vi "Measurement_input_panel.vi"(0 "OK":T4, 2 "setup":T5, 5 "Setup filename":string) -> (11 "Setup filename out":string, 12 "Analysis Info cluster":T8[](array[typedef])=[{"Colour"=0, "Inst type"=enum."Pitot-static tube", "Inst name"="Manometer voltage", "Symbol"="U", "Code name"="", "Extra Info"="U", "Inst Array"=enum."PWA", "Extra Titles"=[], "Extra Values"=[], "U"=0.0, "u^2"=0.0, "u^3"=0.0, "u^4"=0.0, "Skew_u"=0.0, "Kurt_u"=0.0, "Sd Error in Mean"=0.0, "% u'/U"=0.0, "X"=0.0, "Y"=0.0, "Z"=0.0, "Timescale integral to 25%"=0.0, "Sd Error in Variance"=0.0, "Calib File"=path "", "Calib Constants"=[], "Output Position"=FALSE, "Full Stats"=FALSE, "Av Sampling Rate"=0.0, "Av No of Samples"=0.0, "Total Meas Time (s)"=0.0, "ADAM Ch Name"=""}, {"Colour"=0, "Inst type"=enum."Pitot-static tube", "Inst name"="Manometer voltage", "Symbol"="U", "Code name"="", "Extra Info"="U", "Inst Array"=enum."PWA", "Extra Titles"=[], "Extra Values"=[], "U"=0.0, "u^2"=0.0, "u^3"=0.0, "u^4"=0.0, "Skew_u"=0.0, "Kurt_u"=0.0, "Sd Error in Mean"=0.0, "% u'/U"=0.0, "X"=0.0, "Y"=0.0, "Z"=0.0, "Timescale integral to 25%"=0.0, "Sd Error in Variance"=0.0, "Calib File"=path "", "Calib Constants"=[], "Output Position"=FALSE, "Full Stats"=FALSE, "Av Sampling Rate"=0.0, "Av No of Samples"=0.0, "Total Meas Time (s)"=0.0, "ADAM Ch Name"=""}, {"Colour"=0, "Inst type"=enum."Pitot-static tube", "Inst name"="Manometer voltage", "Symbol"="U", "Code name"="", "Extra Info"="U", "Inst Array"=enum."PWA", "Extra Titles"=[], "Extra Values"=[], "U"=0.0, "u^2"=0.0, "u^3"=0.0, "u^4"=0.0, "Skew_u"=0.0, "Kurt_u"=0.0, "Sd Error in Mean"=0.0, "% u'/U"=0.0, "X"=0.0, "Y"=0.0, "Z"=0.0, "Timescale integral to 25%"=0.0, "Sd Error in Variance"=0.0, "Calib File"=path "", "Calib Constants"=[], "Output Position"=FALSE, "Full Stats"=FALSE, "Av Sampling Rate"=0.0, "Av No of Samples"=0.0, "Total Meas Time (s)"=0.0, "ADAM Ch Name"=""}] {"Sd Error in Variance" format="%.2f"; "Skew_u" format="%.2f"; "% u'/U" format="%.2f"; "Sd Error in Mean" format="%.2f"; "Kurt_u" format="%.2f"; "u^4" format="%.2f"; "u^3" format="%.2f"; "U" format="%.2f"; "u^2" format="%.2f"})   [LabVIEW 2013]
uses:
  Controls/Ch_and_spans_choices.ctl
  Controls/Inst_type.ctl
  Controls/Analysis_info_cluster.ctl
  Controls/Instrument_Array.ctl
  Controls/LDA_Setup.ctl
  Controls/Setup.ctl
  Controls/ok_button.ctl
  Controls/Trigger_Mode.ctl
  Controls/PWA_Data.ctl
  File/Setup_Filetype.ctl
  Controls/Post_Process.ctl
  Controls/App_Global.ctl
  Controls/Ch_and_Spans.ctl
  Globals/Meas_global.vi
  Globals/Trav_pos_global.vi
  Globals/LDA_meas_global_1.vi
  Globals/Preference_global.vi
panel:
  in  "Acquisition Plug in":u16(ring) items=["ADAM_Server_Channels.vi", "Channels_and_Index.ctl", "DataTranslation.vi", "DT_With_Multiplexer.vi", "LDA_IP.vi", "NI-DAQmx.vi", "Simulate_kernal.vi"]
  in  "Select Duplicate Channels":bool
  in  "PWA Data":T1
  out "Inst type":T2
  in  "Edit temp and Press":bool
  out "Abs Press (mbar)":dbl=1013.0 format="%.1f"
  out "Temp (deg C)":dbl=21.0 format="%.1f"
  in  "Trigger mode":T3
  in  "Select Plug Ins":bool
  in  "Sync Delay Time (ms)":dbl=24.0 format="%.2f"
  out "XW Present?":bool
  out "Read Setup File?":bool
  out "Setup Paths":string[](array[string])
  in  "Select Local ADAM Channels":bool
  in  "stop":bool
  out "Notes":string
  in  "Setup filename selector":u16(ring) items=["Current_Setup.xls"]
  in  "Synchronise Analogue channels with LDA":bool
  in  "LDA set up":T6={"dimensions"=enum."2D", "Analogue Freq Multiplier"=0.1} {"Analogue Freq Multiplier" min=0.1 max=100.0 format="%_5g"}
  in  "LDA data":enum16{"No LDA data", "Take LDA data"}(ring)=enum."Take LDA data"
  in  "Cross wire":T7(ring)
  in  "No of Analogue inst":i32=1
  in  "Ch & spans choices":T10[](array[typedef]) {"D" format="%.2f"; "Ch No" min=0; "low limit" min=-10 max=10 format="%.2f"; "high limit" min=-10 max=10 format="%.2f"}
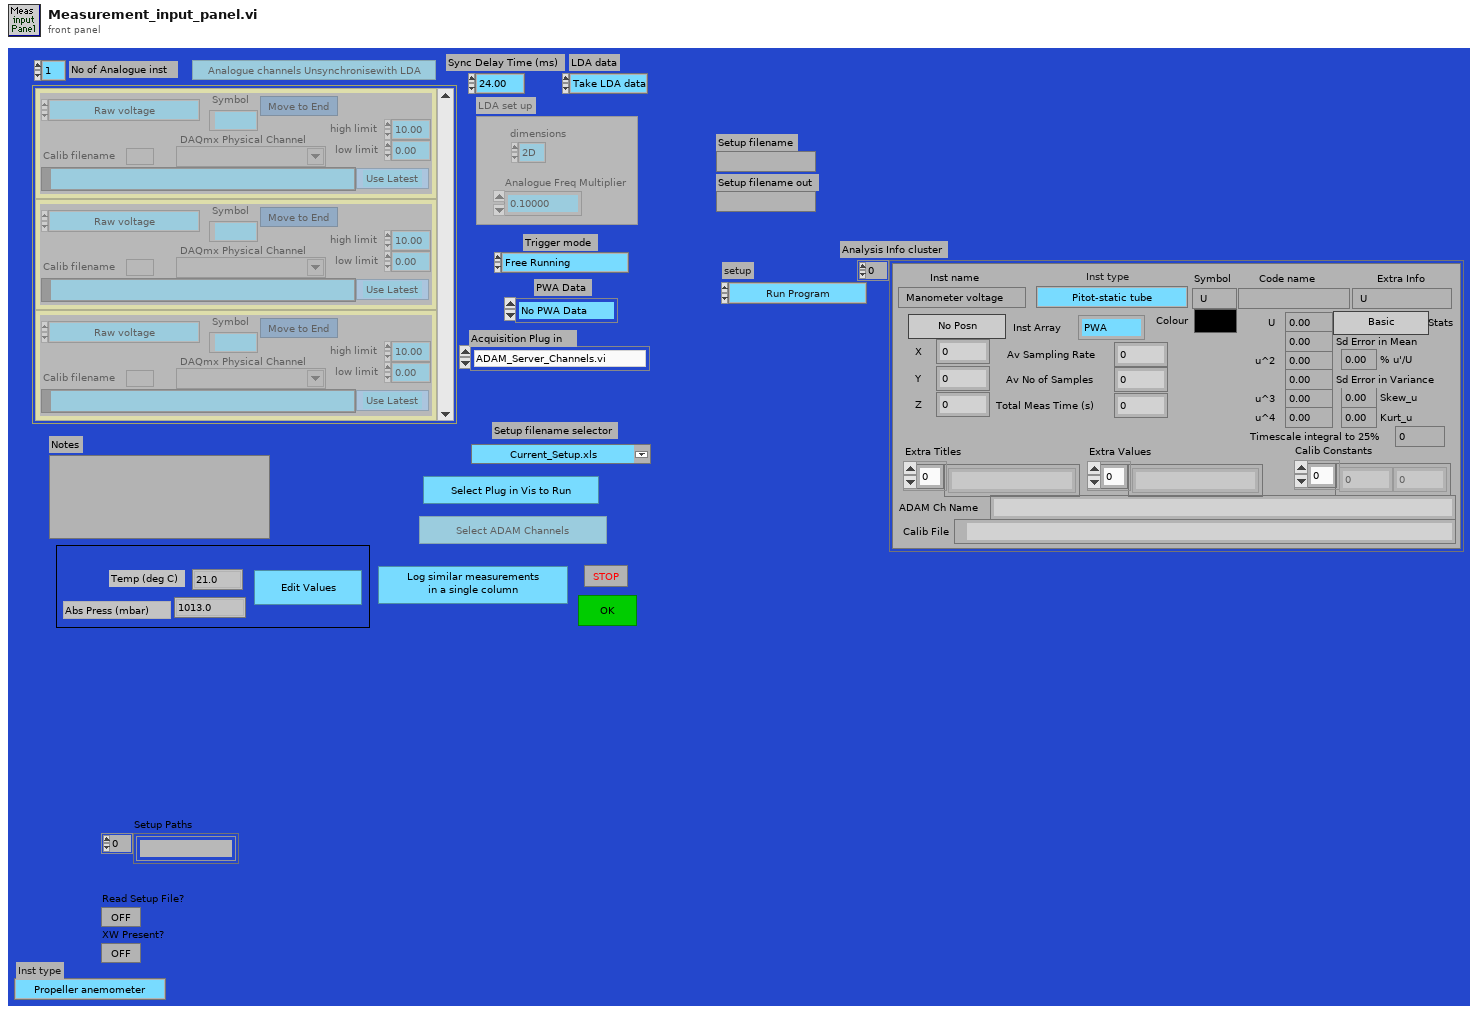
[diagram p1: front panel]
types:
  T1 = typedef "PWA_Data.ctl" = enum16{"No PWA Data", "One Ch PWA"}
  T2 = typedef "Inst_type.ctl" = enum16{"Propeller anemometer", "Raw voltage", "Pressure Transducer", "Pitot-static tube", "Preston tube", "Hot wire", "Cross wire 1", "Cross wire 2", "Generic Linear", "Generic Polynomial", "Generic BackPoly", "Fast FID", "Thermocouple", "Cold wire", "Pulsed Wire", "LDA Vel", "LDA Tran time", "LDA Arr time"}
  T3 = typedef "Trigger_Mode.ctl" = enum16{"Free Running", "Start on Trigger", "Trigger Every Block", "Trigger Every Sample"}
  T4 = typedef "ok_button.ctl" = bool
  T5 = typedef "Setup.ctl" = enum16{"Run Program", "Show Setup", "Save Current Setup", "Setup Front Panel"}
  T6 = typedef "LDA_Setup.ctl" = cluster{"dimensions":enum16{"1D", "2D"}, "Analogue Freq Multiplier":dbl}
  T7 = enum16{"2nd component as calculated", "2nd component multipled by -1"}
  T8 = typedef "Analysis_info_cluster.ctl" = cluster{"Colour":u32, "Inst type":T2, "Inst name":string, "Symbol":string, "Code name":string, "Extra Info":string, "Inst Array":T9, "Extra Titles":string[], "Extra Values":string[], "U":dbl, "u^2":dbl, "u^3":dbl, "u^4":dbl, "Skew_u":dbl, "Kurt_u":dbl, "Sd Error in Mean":dbl, "% u'/U":dbl, "X":dbl, "Y":dbl, "Z":dbl, "Timescale integral to 25%":dbl, "Sd Error in Variance":dbl, "Calib File":path, "Calib Constants":dbl[], "Output Position":bool, "Full Stats":bool, "Av Sampling Rate":dbl, "Av No of Samples":dbl, "Total Meas Time (s)":dbl, "ADAM Ch Name":string}
  T9 = typedef "Instrument_Array.ctl" = enum16{"PWA", "LDA", "Analogue"}
  T10 = typedef "Ch_and_spans_choices.ctl" = cluster{"high limit":sgl, "low limit":sgl, "Ch No":i16, "Calib filename":path, "Inst type":T2, "Symbol":string, "Move channel":bool, "Use Latest":bool, "D":dbl, "Ch Name":string, "DAQmx Physical Channel":tag}
  T11 = typedef "Post_Process.ctl" = enum16{"Take New Data", "Post Process Raw Data File"}
  T12 = typedef "Setup_Filetype.ctl" = enum16{"Measurement Setups", "Calibration Setups", "General", "Results File Plotter Setups", "Speed Calib Tweaks"}
  T13 = typedef "App_Global.ctl" = enum16{"Read Global", "Write to Global", "Initialise Array"}
  T14 = typedef "Ch_and_Spans.ctl" = cluster{"high limit (10V)":sgl, "low limit (-10V)":sgl, "Ch No":i16, "Var name":string, "Use Latest Calib":bool, "DAQmx Chan":tag}
  T15 = enum16{"Zero or one", "One", "Zero or more", "One or more"}
  T16 = typedef "Traverse_cluster.ctl" = cluster{"Start X":dbl, "Start Y":dbl, "Start Z":dbl, "End X":dbl, "End Y":dbl, "End Z":dbl, "No. of pts.":i32, "Spacing":T17, "Filename":path, "Tunnel Speed":dbl, "Averaging time (min)":dbl, "Extra Commands":string, "Specific Arguments":string, "Emission Rate (l/min)":dbl, "Trace Gas Concentration (%)":dbl, "Density Ratio":string, "Comments":string, "Row No":i32, "Row Type Selector":T18, "Completion time":string, "Row Duration (mins)":dbl, "No. of Valid pts.":i32, "Meas Setup File":string}
  T17 = typedef "Spacing.ctl" = enum16{"Linear", "Log", "Gauss", "Specified", "N/A"}
  T18 = typedef "Multi_run_mode.ctl" = enum16{"Move Traverse Only", "Set Tunnel Speed Only", "Set Source Only", "Set Measurement Conditions", "Single Measurement", "Vertical Profile", "Lateral Profile", "Longitudinal Profile", "Explore Volume", "Multi-Axis Profile", "Auto Calibrate", "Meas Fast FID Bkgnd", "Check Beam Power", "Scanning Valve Measurement", "Run VI Named:", "Set ADAM Ch", "Wait (minutes)", "Send Message", "Synchronize With:", "Fall Back to this Row", "Turn Off Row Repeating", "Blank Row", "Traverse 3D Volume"}
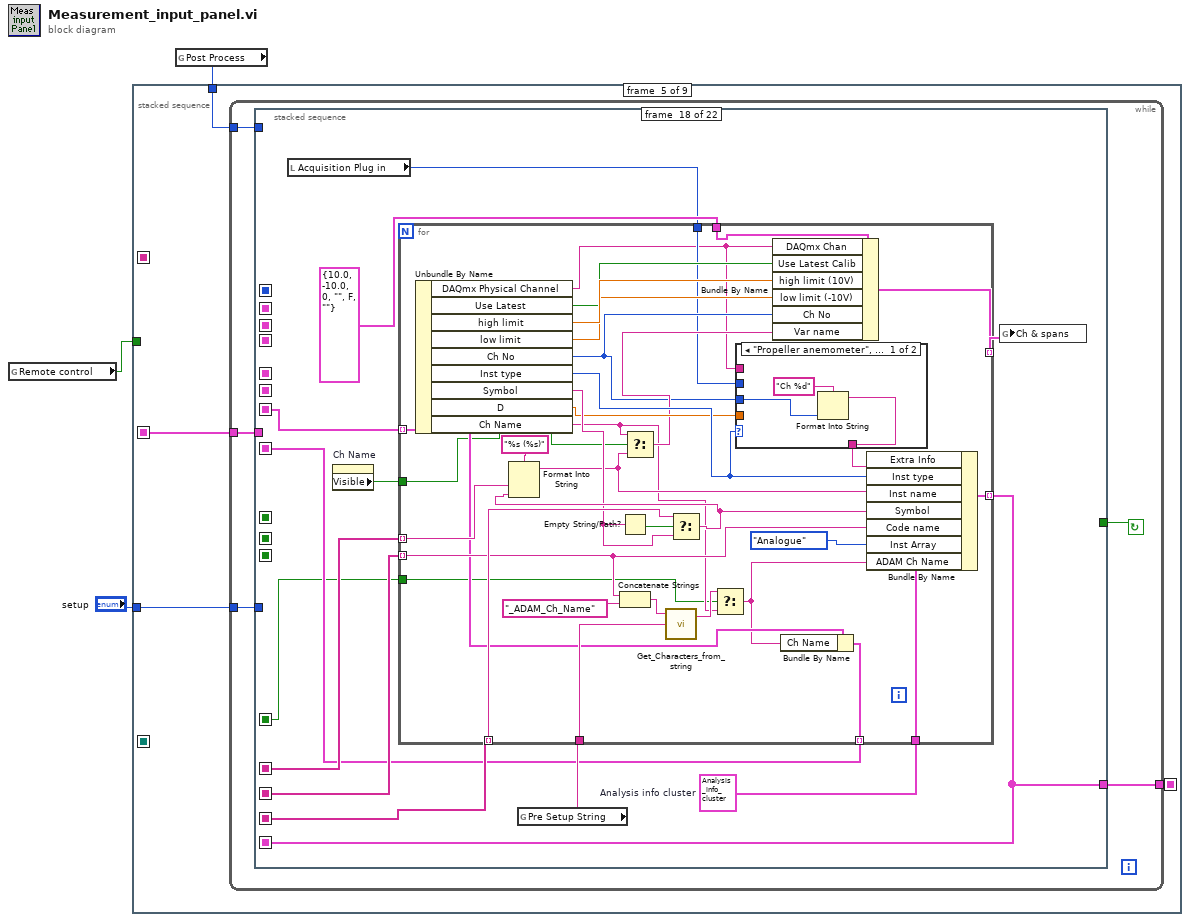
[diagram p0: block diagram]
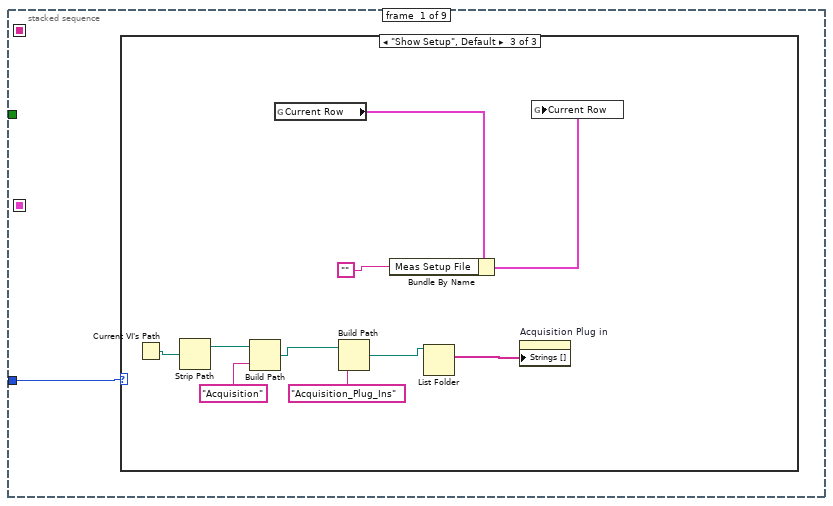
[diagram p2: hidden frame]
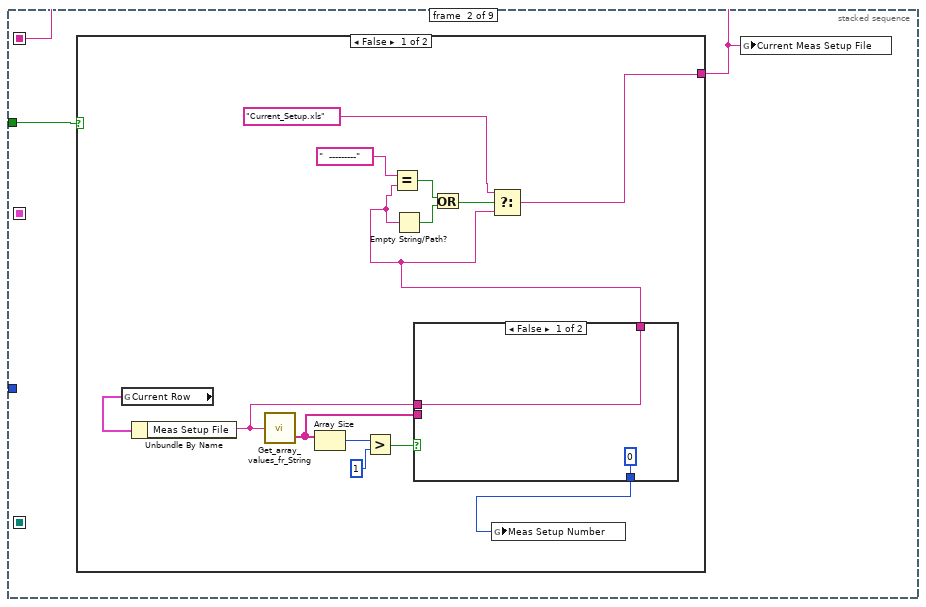
[diagram p5: hidden frame]
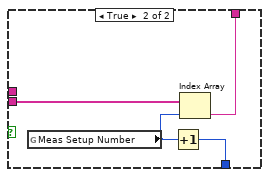
[diagram p6: hidden frame]
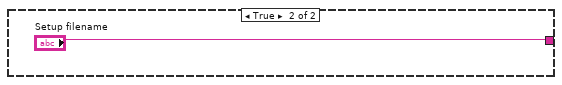
[diagram p7: hidden frame]
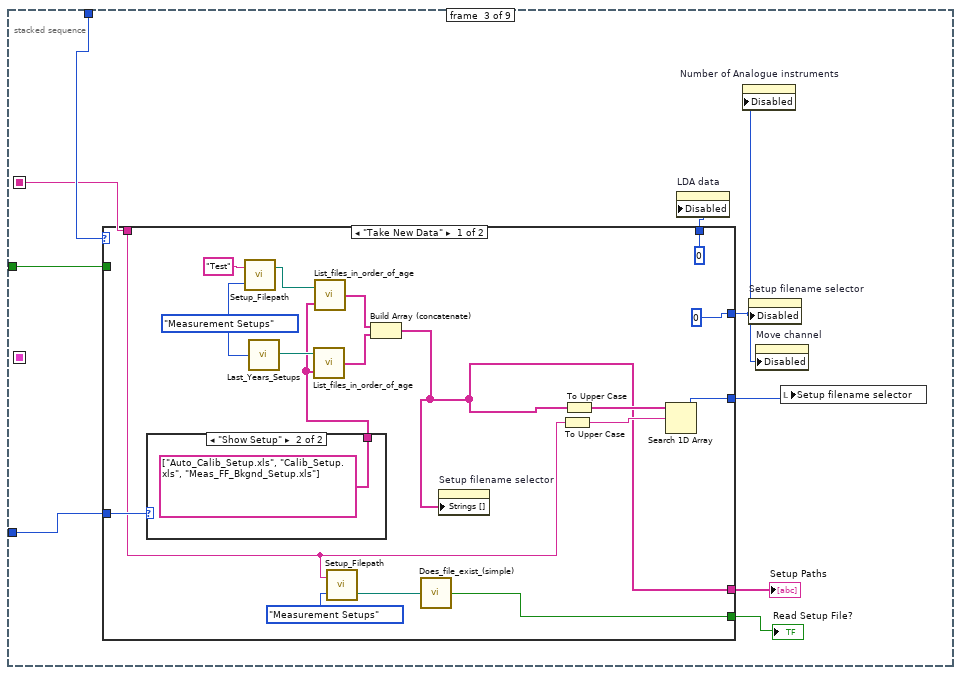
[diagram p8: hidden frame]
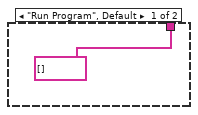
[diagram p9: hidden frame]
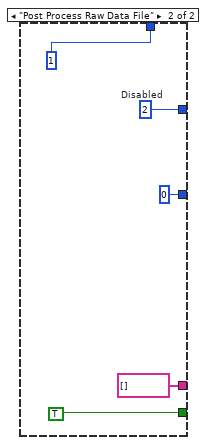
[diagram p10: hidden frame]
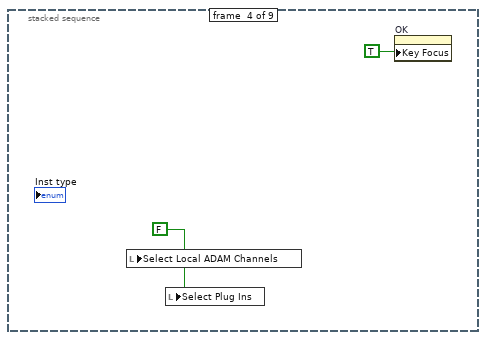
[diagram p11: hidden frame]
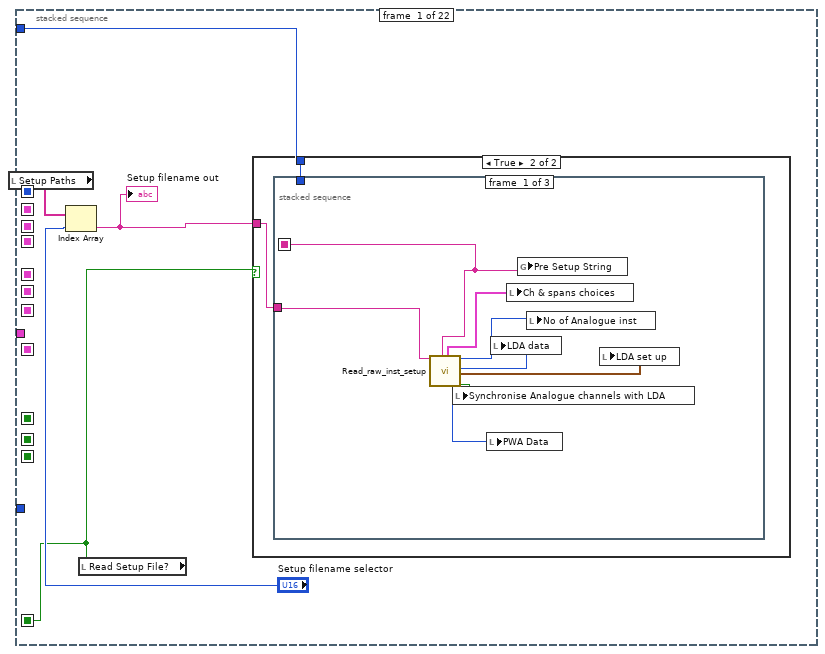
[diagram p12: hidden frame]
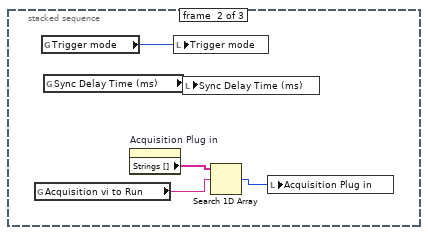
[diagram p14: hidden frame]
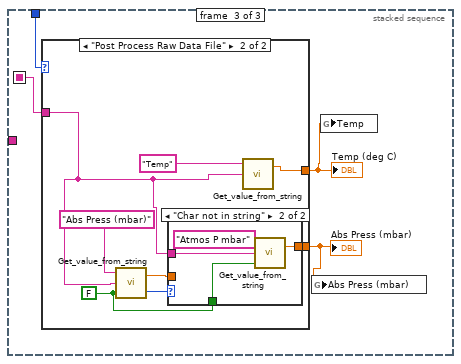
[diagram p15: hidden frame]
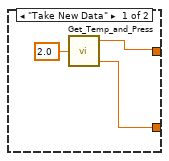
[diagram p16: hidden frame]
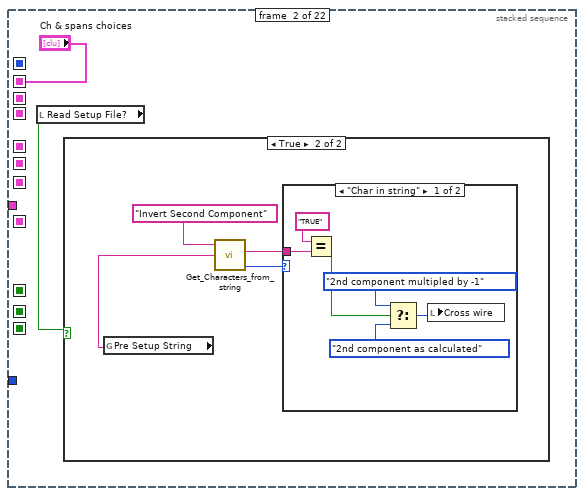
[diagram p18: hidden frame]
diagram:
  n1 = global read "Meas_global.vi" "Remote control"() -> (w1:bool)
  n2 = global read "Meas_global.vi" "Post Process"() -> (w3:T11)
  n3 = stacked-sequence {
    seq-local: [_ _ _ _ w77 _ _ _ _] -> [_ _ _ _ _ _ w720 w821 _]
    seq-local: [_ w15 _ _ _ _ _ _ _] -> [_ _ w38 _ _ _ w719 _ _]
    seq-local: [_ _ _ _ w74 _ _ _ _] -> [_ _ _ _ _ _ _ _ w873]
    seq-local: [_ _ _ _ _ _ _ w820 _] -> [_ _ _ _ _ _ _ _ w872]
    tunnel: w3 -> [_ _ w46 _ w76 _ _ w822 _]
    tunnel: "setup" -> [w4 _ w40 _ w75 _ w721 _ _]
    tunnel: w1 -> [_ w16 w39 _ _ _ _ _ _]
    frame #0 {
      n4 = case shown="\"Show Setup\", Default" w4 {
        frame "Run Program" {
        }
        frame "Setup Front Panel" {
        }
        frame "Show Setup", Default {
          n5 = Current VI's Path() -> (path=w11:path)
          n6 = Strip Path(path=w11) -> (stripped path=w10:path)  [unwired: 1 out]
          n7 = Build Path(base path=w10, name or relative path="Acquisition") -> (appended path=w7:path)
          n8 = global read "Trav_pos_global.vi" "Current Row"() -> (w14:T16)
          n9 = Build Path(base path=w7, name or relative path="Acquisition_Plug_Ins") -> (appended path=w6:path)
          n10 = Bundle By Name(cluster=w14, "Meas Setup File"="") -> (w13:T16)
          n11 = List Folder(path=w6) -> (filenames=w5:string[])  [unwired: 3 in, 3 out]
          n12 = property on="Acquisition Plug in" class="Ring (strict)"("Strings []"=w5) -> ()  [unwired: 2 in, 2 out]
          n13 = global write "Trav_pos_global.vi" "Current Row"(w13) -> ()
        }
      }
    }
    frame #1 {
      n14 = case shown="False" w16 {
        tunnel: [w29 "Setup filename"] -> w15
        frame False {
          n15 = global read "Trav_pos_global.vi" "Current Row"() -> (w25:T16)
          n16 = Unbundle By Name(w25) -> ("Meas Setup File"=w19:string)
          n17 = call "Get_array_values_fr_String.vi"("String Value"=w19) -> ("String array"=w18:string[])  [unwired: 1 out]
          n18 = Array Size(array=w18) -> (size(s)=w23:i32)
          n19 = Greater?(x=w23, y=1) -> (0:w21:bool)
          n20 = case shown="False" w21 {
            tunnel: [w32 w35] -> w20
            tunnel: w19 -> [w32 _]
            tunnel: w18 -> [_ w36]
            tunnel: [0 w33] -> w17
            frame False {
            }
            frame True {
              n21 = global read "Trav_pos_global.vi" "Meas Setup Number"() -> (w34:i32)
              n22 = Increment(x=w34) -> (x+1=w33:i32)
              n23 = Index Array(array=w36, index=w34) -> (element=w35:string)
            }
          }
          n24 = Equal?(x="  ---------" ("f"), y=w20) -> (x = y?=w28:bool)
          n25 = Empty String/Path?(string/path=w20) -> (empty?=w27:bool)
          n26 = Or(x=w28, y=w27) -> (x .or. y?=w24:bool)
          n27 = Select(t="Current_Setup.xls", s=w24, f=w20) -> (s? t:f=w29:string)
          n28 = global write "Trav_pos_global.vi" "Meas Setup Number"(w17) -> ()
        }
        frame True {
        }
      }
      n29 = global write "Trav_pos_global.vi" "Current Meas Setup File"(w15) -> ()
    }
    frame #2 {
      n30 = case shown="\"Take New Data\"" w46 {
        tunnel: [w47 string[] []] -> w42
        tunnel: [w60 TRUE ("exists")] -> w41
        tunnel: [u8 0 ("Disabled") w68] -> w43
        tunnel: [u8 0 ("Disabled") u8 1 ("Disabled")] -> w45
        tunnel: w38 -> [w56 _]
        tunnel: [w63 0 ("index of element")] -> w44
        tunnel: w40 -> [w58 _]
        tunnel: w39 -> [_ _]
        frame "Take New Data" {
          w50 = Setup_Filetype."Measurement Setups" ("Setup File Type")
          n31 = case shown="\"Show Setup\"" w58 {
            tunnel: [string[] [] ("file names") string[] ["Auto_Calib_Setup.xls", "Calib_Setup.xls", "Meas_FF_Bkgnd_Setup.xls"] ("file names")] -> w48
            frame "Run Program", Default {
            }
            frame "Show Setup" {
            }
          }
          n32 = call "Setup_Filepath.vi"("Setup File Type"=w50, "Filename in"="Test") -> ("Directory"=w51:path)  [unwired: 1 out]
          n33 = call "Last_Years_Setups.vi"("Setup File Type"=w50) -> ("Directory"=w49:path)
          n34 = call "List_files_in_order_of_age.vi"("Files to Hide"=w48, "Folder"=w49) -> ("file names"=w53:string[])
          n35 = call "List_files_in_order_of_age.vi"("Files to Hide"=w48, "Folder"=w51) -> ("file names"=w52:string[])
          n36 = call "Setup_Filepath.vi"("Setup File Type"=Setup_Filetype."Measurement Setups", "Filename in"=w56) -> ("Filename Out"=w55:path)  [unwired: 1 out]
          n37 = Build Array (concatenate)(w52, w53) -> (w47:string[])
          n38 = call "Does_file_exist_(simple).vi"("Pathname"=w55) -> ("exists?"=w60:bool)
          n39 = property on="Setup filename selector" class="Ring (strict)"("Strings []"=w47) -> ()  [unwired: 2 in, 2 out]
          n40 = To Upper Case(1:w56) -> (0:w61:string)
          n41 = To Upper Case(1:w47) -> (0:w62:string[])
          n42 = Search 1D Array(1D array=w62, element=w61) -> (index of element=w63:i32)  [unwired: 1 out]
        }
        frame "Post Process Raw Data File" {
          w68 = u8 2  # Disabled
        }
      }
      "Setup Paths" <- w42
      "Read Setup File?" <- w41
      n43 = property on="LDA data" class="Enum (strict)"("Disabled"=w45) -> ()  [unwired: 2 in, 2 out]
      n44 = property on="Number of Analogue instruments" class="DigNum (strict)"("Disabled"=w43) -> ()  [unwired: 2 in, 2 out]
      n45 = property on="Setup filename selector" class="Ring (strict)"("Disabled"=w43) -> ()  [unwired: 2 in, 2 out]
      n46 = property on="Move channel" class="Bool (strict)"("Disabled"=w43) -> ()  [unwired: 2 in, 2 out]
      n47 = local write "Setup filename selector"(w44) -> ()
    }
    frame #3 {
      w73 = FALSE ("Select Local ADAM Channels")
      n48 = local write "Select Local ADAM Channels"(w73) -> ()
      n49 = local write "Select Plug Ins"(w73) -> ()
      n50 = property on="OK" class="Bool"("Key Focus"=TRUE) -> ()  [unwired: 2 in, 2 out]
    }
    frame #4 {
      n51 = while {
        tunnel: w75 -> [w79]
        tunnel: w76 -> [w80]
        tunnel: [w82] -> w77
        tunnel: [w78] -> w74
        stop <- w81 continue-if-true
        n52 = stacked-sequence {
          seq-local: [_ _ _ _ _ _ _ _ _ w242 _ _ _ _ _ _ _ _ _ _ _ _] -> [_ _ _ _ _ _ _ _ _ _ _ w305 w350 w415 _ _ _ _ _ _ _ _]
          seq-local: [_ _ _ _ w166 _ _ _ _ _ _ _ _ _ _ _ _ _ _ _ _ _] -> [_ _ _ _ _ _ w204 _ w238 w243 _ _ _ _ _ _ _ _ _ _ _ _]
          seq-local: [_ _ _ _ _ _ w209 _ _ _ _ _ _ _ _ _ _ _ _ _ _ _] -> [_ _ _ _ _ _ _ _ _ w244 _ _ _ _ _ _ _ _ _ _ _ _]
          seq-local: [_ _ _ _ _ _ _ _ _ _ _ w307 _ _ _ _ _ _ _ _ _ _] -> [_ _ _ _ _ _ _ _ _ _ _ _ w352 _ _ _ _ _ _ _ _ w685]
          seq-local: [_ _ _ _ _ _ _ _ _ _ _ _ _ _ w448 _ _ _ _ _ _ _] -> [_ _ _ _ _ _ _ _ _ _ _ _ _ _ _ w467 _ _ _ _ _ _]
          seq-local: [_ _ _ _ _ _ _ _ _ _ _ _ _ _ _ w463 _ _ _ _ _ _] -> [_ _ _ _ _ _ _ _ _ _ _ _ _ _ _ _ w491 w559 _ _ w661 w686]
          seq-local: [_ _ _ _ _ _ _ _ _ _ _ _ w356 _ _ _ _ _ _ _ _ _] -> [_ _ _ _ _ _ _ _ _ _ _ _ _ _ w445 _ _ _ _ _ _ _]
          seq-local: [_ _ _ _ _ _ _ _ _ _ _ _ _ w419 _ _ _ _ _ _ _ _] -> [_ _ _ _ _ _ _ _ _ _ _ _ _ _ w444 _ _ _ _ _ _ _]
          seq-local: [_ _ _ _ _ _ _ _ _ _ w302 _ _ _ _ _ _ _ _ _ _ _] -> [_ _ _ _ _ _ _ _ _ _ _ w306 w353 _ _ _ _ _ _ _ _ w684]
          seq-local: [_ _ _ _ _ _ _ _ _ _ _ _ _ _ _ _ w490 _ _ _ _ _] -> [_ _ _ _ _ _ _ _ _ _ _ _ _ _ _ _ _ w562 _ _ _ _]
          seq-local: [_ _ _ _ _ _ _ _ _ _ _ _ _ _ _ _ w489 _ _ _ _ _] -> [_ _ _ _ _ _ _ _ _ _ _ _ _ _ _ _ _ w561 _ _ _ _]
          seq-local: [_ _ _ _ _ _ _ _ _ _ _ _ _ _ _ _ w488 _ _ _ _ _] -> [_ _ _ _ _ _ _ _ _ _ _ _ _ _ _ _ _ w560 _ _ _ _]
          seq-local: [_ _ _ _ _ _ _ _ _ _ _ _ _ _ _ _ _ w558 _ _ _ _] -> [_ _ _ _ _ _ _ _ _ _ _ _ _ _ _ _ _ _ _ w611 _ _]
          seq-local: [_ "Ch & spans choices" _ _ _ _ _ _ _ _ _ _ _ _ _ _ _ _ _ _ _ _] -> [_ _ _ _ w155 _ _ _ _ _ _ _ _ _ _ _ _ _ w606 _ _ _]
          seq-local: [_ _ _ _ _ _ _ _ _ _ _ _ _ _ _ _ _ w556 _ _ _ _] -> [_ _ _ _ _ _ _ _ _ _ _ _ _ _ _ _ _ _ w605 _ _ _]
          seq-local: [w83 _ _ _ _ _ _ _ _ _ _ _ _ _ _ _ _ _ _ _ _ _] -> [_ _ _ _ _ _ _ _ _ _ _ _ _ _ _ _ _ w555 _ _ _ _]
          tunnel: [_ _ _ _ _ _ _ _ _ _ _ _ _ _ _ w463 _ _ _ _ _ _] -> w82
          tunnel: [_ _ _ _ _ _ _ _ _ _ _ _ w354 _ _ _ _ _ _ _ _ _] -> w81
          tunnel: w80 -> [w85 _ _ w139 w162 _ _ _ _ _ w303 _ w351 _ w447 _ _ _ _ _ w662 _]
          tunnel: w79 -> [_ _ w135 _ _ w190 _ _ _ _ _ _ _ _ w446 _ _ _ _ w613 _ _]
          tunnel: [_ _ _ _ _ _ _ _ _ _ _ _ _ _ _ _ _ w558 _ _ _ _] -> w78
          frame #0 {
            n53 = local read "Setup Paths"() -> (w87:string[])
            n54 = Index Array(array=w87, index="Setup filename selector") -> (element=w84:string)
            "Setup filename out" <- w84
            n55 = local read "Read Setup File?"() -> (w83:bool)
            n56 = case shown="True" w83 {
              tunnel: w84 -> [_ w89]
              tunnel: w85 -> [_ w88]
              frame False {
              }
              frame True {
                n57 = stacked-sequence {
                  seq-local: [w92 _ _] -> [_ _ w105]
                  tunnel: w89 -> [w94 _ _]
                  tunnel: w88 -> [_ _ w106]
                  frame #0 {
                    n58 = call "Read_raw_inst_setup.vi"("Setup file"=w94) -> ("Setup string"=w92:string, "Ch & spans choices"=w91:T10[], "PWA Data"=w90:T1, "Number of Analogue instruments"=w97:i32, "LDA data"=w96:enum16{"No LDA data", "Take LDA data"}, "LDA set up"=w93:T6, "Synchronise Analogue channels with LDA"=w95:bool)  [unwired: 12 out]
                    n59 = local write "Synchronise Analogue channels with LDA"(w95) -> ()
                    n60 = local write "PWA Data"(w90) -> ()
                    n61 = local write "LDA data"(w96) -> ()
                    n62 = local write "Ch & spans choices"(w91) -> ()
                    n63 = global write "Meas_global.vi" "Pre Setup String"(w92) -> ()
                    n64 = local write "No of Analogue inst"(w97) -> ()
                    n65 = local write "LDA set up"(w93) -> ()
                  }
                  frame #1 {
                    n66 = global read "Meas_global.vi" "Acquisition vi to Run"() -> (w99:string)
                    n67 = global read "Meas_global.vi" "Trigger mode"() -> (w101:T3)
                    n68 = global read "LDA_meas_global_1.vi" "Sync Delay Time (ms)"() -> (w102:dbl)
                    n69 = property on="Acquisition Plug in" class="Ring (strict)"() -> ("Strings []"=w100:string[])  [unwired: 2 in, 2 out]
                    n70 = local write "Trigger mode"(w101) -> ()
                    n71 = local write "Sync Delay Time (ms)"(w102) -> ()
                    n72 = Search 1D Array(1D array=w100, element=w99) -> (index of element=w98:i32)  [unwired: 1 in]
                    n73 = local write "Acquisition Plug in"(w98) -> ()
                  }
                  frame #2 {
                    n74 = case shown="\"Post Process Raw Data File\"" w106 {
                      tunnel: w105 -> [_ w112]
                      tunnel: [w107 w111] -> w103
                      tunnel: [w108 w110] -> w104
                      frame "Take New Data" {
                        n75 = call "Get_Temp_and_Press.vi"("Averaging time (mins)"=2.0) -> ("Abs Press (mbar)"=w107:dbl, "Temperature"=w108:dbl)  [unwired: 3 out]
                      }
                      frame "Post Process Raw Data File" {
                        w114 = FALSE ("Show Dialog?")
                        n76 = call "Get_value_from_string.vi"("Show Dialog?"=w114, "Input string"=w112, "Variable name"="Abs Press (mbar)") -> ("Status"=w116:enum16{"Char in string", "Char not in string"}, "Value"=w115:dbl)
                        n77 = case shown="\"Char not in string\"" w116 {
                          tunnel: [w118 w121] -> w111
                          tunnel: w115 -> [w118 _]
                          tunnel: w114 -> [_ w120]
                          tunnel: w112 -> [_ w119]
                          frame "Char in string" {
                          }
                          frame "Char not in string" {
                            n78 = call "Get_value_from_string.vi"("Show Dialog?"=w120, "Input string"=w119, "Variable name"="Atmos P mbar") -> ("Value"=w121:dbl)  [unwired: 1 out]
                          }
                        }
                        n79 = call "Get_value_from_string.vi"("Input string"=w112, "Variable name"="Temp") -> ("Value"=w110:dbl)  [unwired: 1 in, 1 out]
                      }
                    }
                    "Abs Press (mbar)" <- w103
                    "Temp (deg C)" <- w104
                    n80 = global write "Meas_global.vi" "Abs Press (mbar)"(w103) -> ()
                    n81 = global write "Meas_global.vi" "Temp"(w104) -> ()
                  }
                }
              }
            }
          }
          frame #1 {
            n82 = local read "Read Setup File?"() -> (w124:bool)
            n83 = case shown="True" w124 {
              frame False {
              }
              frame True {
                n84 = global read "Meas_global.vi" "Pre Setup String"() -> (w127:string)
                n85 = call "Get_Characters_from_string.vi"("Input string"=w127, "Variable name"="Invert Second Component") -> ("Status"=w126:enum16{"Char in string", "Char not in string"}, "Value"=w125:string)  [unwired: 1 in]
                n86 = case shown="\"Char in string\"" w126 {
                  tunnel: w125 -> [w134 _]
                  frame "Char in string" {
                    n87 = Equal?(x="TRUE", y=w134) -> (x = y?=w130:bool)
                    n88 = Select(t=T7."2nd component multipled by -1" ("Cross wire/LDA"), s=w130, f=T7."2nd component as calculated" ("Cross wire/LDA")) -> (s? t:f=w132:T7)
                    n89 = local write "Cross wire"(w132) -> ()
                  }
                  frame "Char not in string" {
                  }
                }
              }
            }
          }
          frame #2 {
            n90 = case shown="\"Show Setup\"" w135 {
              frame "Run Program", Default {
              }
              frame "Show Setup" {
                n91 = property on="Acquisition Plug in" class="Ring (strict)"() -> ("Strings []"=w138:string[])  [unwired: 2 in, 2 out]
                n92 = Index Array(array=w138, index="Acquisition Plug in") -> (element=w136:string)
                n93 = global write "Meas_global.vi" "Acquisition vi to Run"(w136) -> ()
              }
            }
          }
          frame #3 {
            n94 = case shown="True" "Edit temp and Press" {
              tunnel: w139 -> [_ w141]
              frame False {
              }
              frame True {
                n95 = case shown="\"Take New Data\"" w141 {
                  frame "Take New Data" {
                    n96 = stacked-sequence {
                      frame #0 {
                        w142 = TRUE  # Wait until done
                        n97 = call "Run_Enter_Temp.vi"("Wait until done"=w142) -> ()  [unwired: 1 out]
                      }
                      frame #1 {
                        n98 = call "Get_Temp_and_Press.vi"("Averaging time (mins)"=2.0) -> ("Abs Press (mbar)"=w143:dbl, "Temperature"=w144:dbl)  [unwired: 3 out]
                        n99 = local write "Temp (deg C)"(w144) -> ()
                        n100 = local write "Abs Press (mbar)"(w143) -> ()
                      }
                    }
                  }
                  frame "Post Process Raw Data File" {
                  }
                }
              }
            }
          }
          frame #4 {
            w158 = u8 0  # Disabled
            n101 = local read "Read Setup File?"() -> (w154:bool)
            n102 = global read "Meas_global.vi" "Acquisition vi to Run"() -> (w149:string)
            n103 = Equal?(x=w162, y=Post_Process."Take New Data" ("Post Process")) -> (x = y?=w161:bool)
            n104 = Equal?(x="ADAM_Server_Channels.vi", y=w149) -> (x = y?=w152:bool)
            n105 = And(x=w154, y=w152) -> (x .and. y?=w165:bool)
            n106 = Or(x="Select Local ADAM Channels", y=w165) -> (x .or. y?=w159:bool)
            n107 = And(x=w161, y=w159) -> (x .and. y?=w160:bool)
            n108 = case shown="True" w160 {
              tunnel: [w167 w168] -> w166
              tunnel: w155 -> [w167 w171]
              tunnel: "Select Local ADAM Channels" -> [_ w170]
              tunnel: w152 -> [_ w169]
              frame False {
              }
              frame True {
                n109 = stacked-sequence {
                  seq-local: [w172 _ _] -> [_ w182 _]
                  tunnel: w171 -> [w174 w181 _]
                  tunnel: [_ w179 _] -> w168
                  tunnel: w170 -> [w176 _ w188]
                  tunnel: w169 -> [w175 _ _]
                  frame #0 {
                    n110 = Array Size(array=w174) -> ()  [unwired: 1 out]
                    n111 = for {
                      tunnel: w174 -> [w178] mode=indexing
                      tunnel: [w177] -> w173 mode=indexing
                      n112 = Unbundle By Name(w178) -> ("Ch Name"=w177:string)
                    }
                    n113 = call "Get_local_ADAM_Chs.vi"("Local ADAM?"=w175, "Show setup"=w176, "Desired Local ADAM Channels"=w173) -> ("Choosen Channels"=w172:string[])  [unwired: 1 out]
                  }
                  frame #1 {
                    n114 = for {
                      tunnel: [w187] -> w179 mode=indexing
                      tunnel: w182 -> [w185]
                      tunnel: w181 -> [w186] mode=indexing
                      i -> [w183]
                      n115 = Index Array(array=w185, index=w183) -> (element=w184:string)
                      n116 = Bundle By Name(cluster=w186, "Ch No"=w183, "Ch Name"=w184) -> (w187:T10)
                    }
                    n117 = Array Size(array=w179) -> (size(s)=w180:i32)
                    n118 = local write "No of Analogue inst"(w180) -> ()
                  }
                  frame #2 {
                    n119 = case shown="True" w188 {
                      frame False {
                      }
                      frame True {
                        n120 = local write "Select Local ADAM Channels"(FALSE ("Select Local ADAM Channels")) -> ()
                      }
                    }
                  }
                }
              }
            }
            n121 = Equal?(x=w149, y="NI-DAQmx.vi") -> (x = y?=w147:bool)
            n122 = Select(t=w158, s=w152, f=u8 2 ("Disabled")) -> (s? t:f=w156:u8)
            n123 = property on="Ch Name" class="Str"("Visible"=w152) -> ()  [unwired: 2 in, 2 out]
            n124 = property on="Select Local ADAM Channels" class="Bool (strict)"("Disabled"=w156) -> ()  [unwired: 2 in, 2 out]
            n125 = Not(x=w152) -> (.not. x?=w151:bool)
            n126 = property on="high limit" class="DigNum (strict)"("Visible"=w151) -> ()  [unwired: 2 in, 2 out]
            n127 = property on="low limit" class="DigNum (strict)"("Visible"=w151) -> ()  [unwired: 2 in, 2 out]
            n128 = property on="Ch No" class="DigNum (strict)"("Visible"=w151) -> (error out=w148:errorcluster)  [unwired: 2 in, 1 out]
            n129 = property on="DAQmx Physical Channel" class="DAQmxName"("Visible"=w147) -> ()  [unwired: 2 in, 2 out]
            n130 = Not(x=w147) -> (.not. x?=w146:bool)
            n131 = property on="Ch No" class="DigNum (strict)"(error in=w148, "Visible"=w146) -> ()  [unwired: 1 in, 2 out]
          }
          frame #5 {
            n132 = case shown="True" "Select Plug Ins" {
              tunnel: w190 -> [_ w192]
              frame False {
              }
              frame True {
                n133 = stacked-sequence {
                  tunnel: w192 -> [w193 _]
                  frame #0 {
                    w197 = TRUE  # Show Panel?
                    n134 = global read "Meas_global.vi" "Pre Setup String"() -> (w196:string)
                    n135 = local write "Select Plug Ins"(FALSE ("Select Local ADAM Channels")) -> ()
                    n136 = call "Choose_Plug_In_to_Run.vi"("setup"=w193, "Show Panel?"=w197, "Setup String In"=w196) -> ("Setup String Out"=w195:string)  [unwired: 1 out]
                    n137 = global write "Meas_global.vi" "Pre Setup String"(w195) -> ()
                  }
                  frame #1 {
                    n138 = Current VI's Path() -> (path=w199:path)
                    n139 = call "Open_Close_Front_Panel.ph.vi"("Front Panel Window:Open"=TRUE, "VI path"=w199) -> ()  [unwired: 2 out]
                  }
                }
              }
            }
          }
          frame #6 {
            n140 = Initialize Array(0) -> (w211:i32[])  [unwired: 1 out]
            n141 = for {
              shift-right: [w218] -> w207
              shift-left: w211 -> [w219]
              tunnel: [w217] -> w205 mode=indexing
              tunnel: w204 -> [w216] mode=indexing
              tunnel: [w214] -> w203 mode=indexing
              n142 = Unbundle By Name(w216) -> ("Inst type"=w213:T2)
              n143 = case shown="\"Cross wire 2\"" w213 {
                tunnel: w219 -> [w223 w227 w229 w233]
                tunnel: [w222 w226 w229 w232] -> w218
                tunnel: [FALSE TRUE FALSE FALSE] -> w217
                frame "Propeller anemometer", Default {
                  n144 = Build Array (concatenate)(w223, 1) -> (w222:i32[])
                }
                frame "Cross wire 1" {
                  n145 = Build Array (concatenate)(w227, 2) -> (w226:i32[])
                }
                frame "Cross wire 2" {
                }
                frame "LDA Vel" {
                  n146 = Build Array (concatenate)(w233, 1) -> (w232:i32[])
                }
              }
              n147 = Equal?(x=w213, y=Inst_type."Preston tube" ("Inst type")) -> (x = y?=w214:bool)
            }
            n148 = Build Array (concatenate)(w207, 1) -> (w206:i32[])
            n149 = Array Subset(array=w206, length="No of Analogue inst") -> (w210:i32[])  [unwired: 1 in]
            n150 = Add Array Elements(numeric array=w210) -> (sum=w209:i32)
            n151 = Or Array Elements(Boolean array=w205) -> (logical OR=→"XW Present?":bool)
            n152 = Or Array Elements(Boolean array=w203) -> (logical OR=w201:bool)
            n153 = property on="D" class="DigNum (strict)"("Visible"=w201) -> ()  [unwired: 2 in, 2 out]
          }
          frame #7 {
            "Notes" <- ""
          }
          frame #8 {
            n154 = Array Size(array=w238) -> (size(s)=w237:i32)
            n155 = Not Equal To 0?(x=w237) -> (x != 0?=w236:bool)
            n156 = case shown="True" w236 {
              tunnel: [enum16{"No Analogue data", "Take Analogue data"}."No Analogue data" ("Analogue data") enum16{"No Analogue data", "Take Analogue data"}."Take Analogue data" ("Analogue data")] -> w235
              frame False {
              }
              frame True {
              }
            }
            n157 = global write "Meas_global.vi" "Analogue data"(w235) -> ()
          }
          frame #9 {
            n158 = Index Array(array=w243, index=0) -> (element=w248:T10)
            n159 = Initialize Array(w248) -> (w246:T10[])  [unwired: 1 out]
            n160 = Build Array (concatenate)(w243, w248) -> (w247:T10[])
            n161 = for {
              N: w244 -> [_]
              tunnel: w247 -> [w256] mode=indexing
              shift-right: [w257] -> w242
              shift-left: w246 -> [w251]
              tunnel: Inst_type."Cross wire 2" ("Inst type") -> [w249]
              shift-right: [w255] -> _
              shift-left: _ -> [w254]
              tunnel: w247 -> [w253]
              n162 = Unbundle By Name(w256) -> ("Inst type"=w255:T2)
              n163 = Array Size(array=w251) -> (size(s)=w250:i32)
              n164 = Increment(x=w250) -> (x+1=w252:i32)
              n165 = case shown="\"Cross wire 2\"" w255 {
                tunnel: [w266 w287 w299] -> w257
                tunnel: w251 -> [w267 w289 w301]
                tunnel: w256 -> [w263 w290 w300]
                tunnel: w249 -> [w265 w294 _]
                tunnel: w254 -> [_ w293 _]
                tunnel: w253 -> [w270 _ _]
                tunnel: w252 -> [w269 _ _]
                frame "Cross wire 1" {
                  n166 = Index Array(array=w270, index=w269) -> (element=w264:T10)
                  n167 = Unbundle By Name(w264) -> ("Inst type"=w268:T2, "high limit"=w261:sgl, "low limit"=w260:sgl, "Ch No"=w259:i16, "Symbol"=w258:string)
                  n168 = Unbundle By Name(w263) -> ("Calib filename"=w262:path)
                  n169 = case shown="\"Cross wire 2\"" w268 {
                    tunnel: w267 -> [w280 w286]
                    tunnel: [w279 w285] -> w266
                    tunnel: w265 -> [w272 w281]
                    tunnel: w262 -> [w278 w284]
                    tunnel: w263 -> [w276 w282]
                    tunnel: w264 -> [_ _]
                    tunnel: w261 -> [w275 _]
                    tunnel: w260 -> [w274 _]
                    tunnel: w259 -> [w273 _]
                    tunnel: w258 -> [w271 _]
                    frame "Cross wire 2" {
                      n170 = Bundle By Name(cluster=w276, "Calib filename"=w278, "Inst type"=w272, "high limit"=w275, "low limit"=w274, "Ch No"=w273, "Symbol"=w271) -> (w277:T10)
                      n171 = Build Array (concatenate)(w280, w276, w277) -> (w279:T10[])
                    }
                    frame "Generic Linear", Default {
                      n172 = Bundle By Name(cluster=w282, "Calib filename"=w284, "Inst type"=w281) -> (w283:T10)
                      n173 = Build Array (concatenate)(w286, w282, w283) -> (w285:T10[])
                    }
                  }
                }
                frame "Cross wire 2" {
                  n174 = Decrement(x=w294) -> (x-1=w292:T2)
                  n175 = Equal?(x=w292, y=w293) -> (x = y?=w291:bool)
                  n176 = Bundle By Name(cluster=w290, "Inst type"=w292) -> (w288:T10)
                  n177 = case shown="False" w291 {
                    tunnel: w290 -> [_ _]
                    tunnel: w289 -> [w297 w298]
                    tunnel: w288 -> [w296 _]
                    tunnel: [w295 w298] -> w287
                    frame False {
                      n178 = Build Array (concatenate)(w297, w296) -> (w295:T10[])
                    }
                    frame True {
                    }
                  }
                }
                frame "Generic Linear", Default {
                  n179 = Build Array (concatenate)(w301, w300) -> (w299:T10[])
                }
              }
            }
          }
          frame #10 {
            n180 = Equal?(x=w303, y=Post_Process."Take New Data" ("Post Process")) -> (x = y?=w302:bool)
          }
          frame #11 {
            n181 = case shown="True" "OK" {
              tunnel: w305 -> [_ w322]
              tunnel: [FALSE w321] -> w307
              tunnel: w306 -> [_ w310]
              frame False {
              }
              frame True {
                n182 = for {
                  tunnel: w322 -> [w334] mode=indexing
                  tunnel: [w332] -> w316 mode=indexing
                  tunnel: [w328] -> w320 mode=indexing
                  n183 = Unbundle By Name(w334) -> ("high limit"=w337:sgl, "low limit"=w336:sgl, "Ch No"=w333:i16, "Inst type"=w331:T2, "Symbol"=w330:string)
                  n184 = Number To Decimal String(number=w331) -> (decimal integer string=w329:string)  [unwired: 1 out]
                  n185 = Concatenate Strings(w329, w330) -> (w328:string)
                  n186 = Greater Or Equal?(x=w337, y=w336) -> (x >= y?=w335:bool)
                  n187 = case shown="\"Propeller anemometer\", Default" w331 {
                    tunnel: w335 -> [w340 _ _ _]
                    tunnel: w333 -> [w339 _ _ _]
                    tunnel: [w338 TRUE TRUE TRUE] -> w332
                    frame "Propeller anemometer", Default {
                      n188 = case shown="False" w340 {
                        tunnel: w339 -> [w343 _]
                        tunnel: [FALSE TRUE] -> w338
                        frame False {
                          n189 = Number To Decimal String(number=w343) -> (decimal integer string=w342:string)  [unwired: 1 out]
                          n190 = Concatenate Strings("Error in input limits for Channel No ", w342) -> (w344:string)
                          n191 = One Button Dialog(message=w344) -> ()  [unwired: 2 out]
                        }
                        frame True {
                        }
                      }
                    }
                    frame "LDA Vel" {
                    }
                    frame "LDA Tran time" {
                    }
                    frame "LDA Arr time" {
                    }
                  }
                }
                n192 = call "Analyse_string_array.vi"("String array"=w320) -> ("Frequency"=w319:i32[])  [unwired: 2 out]
                n193 = global read "Meas_global.vi" "Remote control"() -> (w311:bool)
                n194 = Greater?(x=w319, y=1) -> (0:w317:bool[])
                n195 = Or Array Elements(Boolean array=w317) -> (logical OR=w313:bool)
                n196 = Compound Arithmetic op=AND(invert w311, w313, w310) -> (w312:bool)
                n197 = case shown="True" w312 {
                  tunnel: [TRUE FALSE] -> w315
                  frame False {
                  }
                  frame True {
                    n198 = Current VI's Path() -> (path=w325:path)
                    n199 = call "Open_Close_Front_Panel.ph.vi"("Front Panel Window:Open"=TRUE, "VI path"=w325) -> ()  [unwired: 2 out]
                    n200 = One Button Dialog(message="Non Unique symbol names") -> ()  [unwired: 2 out]
                  }
                }
                n201 = Build Array (concatenate)(w316, w315) -> (w314:bool[])
                n202 = And Array Elements(Boolean array=w314) -> (logical AND=w321:bool)
              }
            }
          }
          frame #12 {
            n203 = And(x=w353, y=w352) -> (x .and. y?=w355:bool)
            n204 = case shown="True" w355 {
              tunnel: w350 -> [_ w364]
              tunnel: [FALSE w363] -> w356
              tunnel: [w357 w362] -> w354
              tunnel: w352 -> [w358 _]
              tunnel: w351 -> [_ _]
              frame False {
                n205 = Not(x=w358) -> (.not. x?=w357:bool)
              }
              frame True {
                n206 = for {
                  shift-right: [w386] -> _
                  shift-left: i16[] [] -> [w385]
                  tunnel: w364 -> [w369] mode=indexing
                  tunnel: [w374] -> w365 mode=indexing
                  shift-right: [w382] -> _
                  shift-left: path[] [] -> [w381]
                  shift-right: [w368] -> _
                  shift-left: tag[] [] -> [w367]
                  n207 = Unbundle By Name(w369) -> ("Ch No"=w383:i16)
                  n208 = local read "Acquisition Plug in"() -> (w370:u16)
                  n209 = Unbundle By Name(w369) -> ("Inst type"=w380:T2, "Calib filename"=w377:path)
                  n210 = Search 1D Array(1D array=w385, element=w383) -> (index of element=w384:i32)  [unwired: 1 out]
                  n211 = Build Array (concatenate)(w385, w383) -> (w386:i16[])
                  n212 = Equal?(x=Inst_type."Fast FID" ("Inst type"), y=w380) -> (x = y?=w373:bool)
                  n213 = case shown="5" w370 {
                    tunnel: w384 -> [w390 _]
                    tunnel: w383 -> [w389 _]
                    tunnel: [w388 w401] -> w376
                    tunnel: w369 -> [_ w404]
                    tunnel: [w387 w403] -> w368
                    tunnel: w367 -> [w387 w402]
                    frame 0, Default {
                      n214 = case shown="0, Default" w390 {
                        tunnel: w389 -> [w395 _]
                        tunnel: [w391 FALSE ("true")] -> w388
                        frame 0, Default {
                          n215 = Format Into String(format string="The Ch No %d appears more than once", w395) -> (resulting string=w393:string)  [unwired: 2 in, 1 out]
                          n216 = One Button Dialog(message=w393, button name ("OK")="Ok") -> (true=w391:bool)
                        }
                        frame -1 {
                        }
                      }
                    }
                    frame 5 {
                      # "NI-DAQmx"
                      n217 = Unbundle By Name(w404) -> ("DAQmx Physical Channel"=w397:tag)
                      n218 = Search 1D Array(1D array=w402, element=w397) -> (index of element=w400:i32)  [unwired: 1 in]
                      n219 = Format Into String(format string="The Ch %s appears more than once", w397) -> (resulting string=w398:string)  [unwired: 2 in, 1 out]
                      n220 = Build Array (concatenate)(w402, w397) -> (w403:tag[])
                      n221 = case shown="-1" w400 {
                        tunnel: [FALSE ("true") w407] -> w401
                        tunnel: w398 -> [_ w406]
                        frame -1 {
                        }
                        frame 1, Default {
                          n222 = One Button Dialog(message=w406, button name ("OK")="Ok") -> (true=w407:bool)
                        }
                      }
                    }
                  }
                  n223 = Search 1D Array(1D array=w381, element=w377) -> (index of element=w378:i32)  [unwired: 1 out]
                  n224 = Greater Or Equal To 0?(x=w378) -> (x >= 0?=w372:bool)
                  n225 = And(x=w373, y=w372) -> (x .and. y?=w371:bool)
                  n226 = case shown="True" w371 {
                    tunnel: [w410 FALSE ("true")] -> w375
                    tunnel: w377 -> [w409 _]
                    frame True {
                      n227 = Format Into String(format string="Calibration file %s is used more than once.", w409) -> (resulting string=w412:string)  [unwired: 2 in, 1 out]
                      n228 = One Button Dialog(message=w412, button name ("OK")="Ok") -> (true=w410:bool)
                    }
                    frame False {
                    }
                  }
                  n229 = Build Array (concatenate)(w381, w377) -> (w382:path[])
                  n230 = Or(x=w376, y=w375) -> (x .or. y?=w374:bool)
                }
                n231 = Or Array Elements(Boolean array=w365) -> (logical OR=w362:bool)
                n232 = Not(x=w362) -> (.not. x?=w363:bool)
              }
            }
          }
          frame #13 {
            n233 = call "Current_Calib_Filenames.vi"("Mode"=App_Global."Read Global") -> ("Calib Filename Out"=w416:path[], "Channel Numbers Out"=w417:i16[])  [unwired: 2 in, 1 out]
            n234 = for {
              tunnel: w415 -> [w430] mode=indexing
              tunnel: w417 -> [w432]
              tunnel: w416 -> [w431]
              tunnel: [w429] -> w419 mode=indexing
              w427 = Inst_type."Cross wire 2"  # Inst type
              n235 = Unbundle By Name(w430) -> ("Inst type"=w422:T2, "Ch No"=w424:i16, "Use Latest"=w425:bool, "Inst type"=w428:T2)
              n236 = Not Equal?(x=w428, y=w427) -> (x != y?=w426:bool)
              n237 = Compound Arithmetic op=AND(w425, w426) -> (w423:bool)
              n238 = Not Equal?(x=Inst_type."Raw voltage" ("Inst type"), y=w422) -> (x != y?=w420:bool)
              n239 = case shown="True" w423 {
                tunnel: w432 -> [_ w443]
                tunnel: w424 -> [_ w442]
                tunnel: w431 -> [_ w440]
                tunnel: w430 -> [w433 w439]
                tunnel: [w433 w438] -> w429
                tunnel: w420 -> [_ w435]
                frame False {
                }
                frame True {
                  n240 = Search 1D Array(1D array=w443, element=w442) -> (index of element=w441:i32)  [unwired: 1 out]
                  n241 = Index Array(array=w440, index=w441) -> (element=w436:path)
                  n242 = Select(t=w436, s=w435, f=path "") -> (s? t:f=w437:path)
                  n243 = Bundle By Name(cluster=w439, "Calib filename"=w437) -> (w438:T10)
                }
              }
            }
          }
          frame #14 {
            n244 = case shown="True" w445 {
              tunnel: w444 -> [w449 w452]
              tunnel: [w449 w451] -> w448
              tunnel: w447 -> [_ _]
              tunnel: w446 -> [_ w450]
              frame False {
              }
              frame True {
                n245 = case shown="\"Run Program\", Default" w450 {
                  tunnel: w452 -> [w454 w462]
                  tunnel: [w453 w462] -> w451
                  frame "Run Program", Default {
                    n246 = for {
                      tunnel: w454 -> [w455] mode=indexing
                      tunnel: [w456] -> w453 mode=indexing
                      n247 = Unbundle By Name(w455) -> ("Calib filename"=w461:path, "Use Latest"=w460:bool, "Ch No"=w459:i16, "Inst type"=w458:T2)
                      n248 = call "Find_calibration_file.vi"("Inst type"=w458, "Ch No"=w459, "Use Latest Calib"=w460, "filename"=w461) -> ("filename out"=w457:path)
                      n249 = Bundle By Name(cluster=w455, "Calib filename"=w457) -> (w456:T10)
                    }
                  }
                  frame "Setup Front Panel" {
                  }
                }
              }
            }
          }
          frame #15 {
            w465 = 0 ("Index")
            n250 = Index Array(array=w467, index=w465) -> (element=w466:T10)
            n251 = Initialize Array(w466, w465) -> (w464:T10[])
            n252 = for {
              shift-right: [w475] -> w469
              shift-left: w464 -> [w474]
              shift-right: [w476] -> w470
              shift-left: w464 -> [w478]
              tunnel: w467 -> [w477] mode=indexing
              n253 = Unbundle By Name(w477) -> ("Move channel"=w479:bool)
              n254 = case shown="True" w479 {
                tunnel: w478 -> [w481 w487]
                tunnel: w477 -> [w483 w486]
                tunnel: [w482 w487] -> w476
                tunnel: [w480 w485] -> w475
                tunnel: w474 -> [w480 w484]
                frame False {
                  n255 = Build Array (concatenate)(w481, w483) -> (w482:T10[])
                }
                frame True {
                  n256 = Build Array (concatenate)(w484, w486) -> (w485:T10[])
                }
              }
            }
            n257 = Build Array (concatenate)(w470, w469) -> (w468:T10[])
            n258 = for {
              tunnel: w468 -> [w473] mode=indexing
              tunnel: [w471] -> w463 mode=indexing
              n259 = Bundle By Name(cluster=w473, "Move channel"=FALSE) -> (w471:T10)
            }
          }
          frame #16 {
            n260 = for {
              shift-right: [w497] -> _
              shift-left: string[] [] -> [w498]
              tunnel: [w500] -> w489 mode=indexing
              tunnel: [w494] -> w490 mode=indexing
              tunnel: w491 -> [w496] mode=indexing
              tunnel: [w493] -> w488 mode=indexing
              n261 = Unbundle By Name(w496) -> ("Inst type"=w499:T2)
              n262 = case shown="\"Raw voltage\"" w499 {
                tunnel: [w507 w511 w514 w518 w522 w526 w530 "XW" w537 w542 w545 w549] -> w494
                tunnel: ["U" "P" "U" "U" "tau" "U" "U" "W" "U" "C" "T" "T"] -> w501
                tunnel: w498 -> [w508 w512 w516 w520 w524 w528 w532 w534 w539 w543 w547 w551]
                tunnel: [w506 w510 w515 w519 w523 w527 w531 w534 w538 w541 w546 w550] -> w497
                frame "Propeller anemometer" {
                  w507 = "Prop"
                  n263 = Build Array (concatenate)(w508, w507) -> (w506:string[])
                }
                frame "Pressure Transducer" {
                  w511 = "Mano"
                  n264 = Build Array (concatenate)(w512, w511) -> (w510:string[])
                }
                frame "Raw voltage" {
                  w514 = "RV"
                  n265 = Build Array (concatenate)(w516, w514) -> (w515:string[])
                }
                frame "Pitot-static tube" {
                  w518 = "Pitot"
                  n266 = Build Array (concatenate)(w520, w518) -> (w519:string[])
                }
                frame "Preston tube" {
                  w522 = "Preston"
                  n267 = Build Array (concatenate)(w524, w522) -> (w523:string[])
                }
                frame "Hot wire" {
                  w526 = "HW"
                  n268 = Build Array (concatenate)(w528, w526) -> (w527:string[])
                }
                frame "Cross wire 1" {
                  w530 = "XW"
                  n269 = Build Array (concatenate)(w532, w530) -> (w531:string[])
                }
                frame "Cross wire 2" {
                }
                frame "Generic Linear", Default {
                  w537 = "Gen"
                  n270 = Build Array (concatenate)(w539, w537) -> (w538:string[])
                }
                frame "Fast FID" {
                  w542 = "FF"
                  n271 = Build Array (concatenate)(w543, w542) -> (w541:string[])
                }
                frame "Thermocouple" {
                  w545 = "T"
                  n272 = Build Array (concatenate)(w547, w545) -> (w546:string[])
                }
                frame "Cold wire" {
                  w549 = "CW"
                  n273 = Build Array (concatenate)(w551, w549) -> (w550:string[])
                }
              }
              n274 = call "Analyse_string_array.vi"("String array"=w497) -> ("Unique strings"=w505:string[], "Frequency"=w503:i32[])  [unwired: 1 out]
              n275 = Search 1D Array(1D array=w505, element=w494) -> (index of element=w504:i32)  [unwired: 1 out]
              n276 = Index Array(array=w503, index=w504) -> (element=w495:i32)
              n277 = Number To Decimal String(number=w495) -> (decimal integer string=w493:string)  [unwired: 1 out]
              n278 = Concatenate Strings(w493, w494, ":", w501) -> (w500:string)
            }
          }
          frame #17 {
            w564 = T8 {"Colour"=0, "Inst type"=enum."Pitot-static tube", "Inst name"="Manometer voltage", "Symbol"="U", "Code name"="", "Extra Info"="U", "Inst Array"=enum."PWA", "Extra Titles"=[], "Extra Values"=[], "U"=0.0, "u^2"=0.0, "u^3"=0.0, "u^4"=0.0, "Skew_u"=0.0, "Kurt_u"=0.0, "Sd Error in Mean"=0.0, "% u'/U"=0.0, "X"=0.0, "Y"=0.0, "Z"=0.0, "Timescale integral to 25%"=0.0, "Sd Error in Variance"=0.0, "Calib File"=path "", "Calib Constants"=[], "Output Position"=FALSE, "Full Stats"=FALSE, "Av Sampling Rate"=0.0, "Av No of Samples"=0.0, "Total Meas Time (s)"=0.0, "ADAM Ch Name"=""}  # Analysis info cluster
            n279 = local read "Acquisition Plug in"() -> (w553:u16)
            n280 = property on="Ch Name" class="Str"() -> ("Visible"=w565:bool)  [unwired: 2 in, 2 out]
            n281 = global read "Meas_global.vi" "Pre Setup String"() -> (w557:string)
            n282 = for {
              tunnel: [w598] -> w554 mode=indexing
              tunnel: w559 -> [w575] mode=indexing
              tunnel: w562 -> [w590] mode=indexing
              tunnel: T14 {"high limit (10V)"=10.0, "low limit (-10V)"=-10.0, "Ch No"=0, "Var name"="", "Use Latest Calib"=FALSE, "DAQmx Chan"=""} ("Ch and Spans") -> [w595]
              tunnel: [w594] -> w558 mode=indexing
              tunnel: w561 -> [w578] mode=indexing
              tunnel: w564 -> [w592]
              tunnel: w560 -> [w587] mode=indexing
              tunnel: w565 -> [w571]
              tunnel: w557 -> [w579]
              tunnel: [w574] -> w556 mode=indexing
              tunnel: w555 -> [w570]
              tunnel: w553 -> [w568]
              n283 = Unbundle By Name(w575) -> ("DAQmx Physical Channel"=w567:tag, "Use Latest"=w591:bool, "high limit"=w597:sgl, "low limit"=w596:sgl, "Ch No"=w569:i16, "Inst type"=w585:T2, "Symbol"=w584:string, "D"=w583:dbl, "Ch Name"=w572:string)
              n284 = Empty String/Path?(string/path=w584) -> (empty?=w588:bool)
              n285 = Concatenate Strings(w578, "_ADAM_Ch_Name" ("string")) -> (w576:string)
              n286 = call "Get_Characters_from_string.vi"("Input string"=w579, "Variable name"=w576) -> ("Value"=w573:string)  [unwired: 1 in, 1 out]
              n287 = Select(t=w587, s=w588, f=w584) -> (s? t:f=w586:string)
              n288 = Format Into String(format string="%s (%s)" ("Format String"), w590, w586) -> (resulting string=w581:string)  [unwired: 2 in, 1 out]
              n289 = Select(t=w572, s=w571, f=w581) -> (s? t:f=w580:string)
              n290 = Select(t=w573, s=w570, f=w572) -> (s? t:f=w566:string)
              n291 = case shown="\"Propeller anemometer\", Default" w585 {
                tunnel: [w601 w604] -> w593
                tunnel: w569 -> [w600 _]
                tunnel: w583 -> [_ w602]
                tunnel: w568 -> [_ _]
                tunnel: w567 -> [_ _]
                frame "Propeller anemometer", Default {
                  n292 = Format Into String(format string="Ch %d" ("Format String"), w600) -> (resulting string=w601:string)  [unwired: 2 in, 1 out]
                }
                frame "Preston tube" {
                  n293 = Format Into String(format string="D = %.2f" ("Format String"), w602) -> (resulting string=w604:string)  [unwired: 2 in, 1 out]
                }
              }
              n294 = Bundle By Name(cluster=w595, "DAQmx Chan"=w567, "Use Latest Calib"=w591, "high limit (10V)"=w597, "low limit (-10V)"=w596, "Ch No"=w569, "Var name"=w580) -> (w598:T14)
              n295 = Bundle By Name(cluster=w575, "Ch Name"=w566) -> (w574:T10)
              n296 = Bundle By Name(cluster=w592, "Extra Info"=w593, "Inst type"=w585, "Inst name"=w581, "Symbol"=w586, "Code name"=w578, "Inst Array"=Instrument_Array."Analogue", "ADAM Ch Name"=w566) -> (w594:T8)
            }
            n297 = global write "Meas_global.vi" "Ch & spans"(w554) -> ()
          }
          frame #18 {
            n298 = Not Equal?(x=w606, y=w605) -> (x != y?=w607:bool)
            n299 = case shown="True" w607 {
              tunnel: w605 -> [_ w608]
              frame False {
              }
              frame True {
                n300 = local write "Ch & spans choices"(w608) -> ()
              }
            }
          }
          frame #19 {
            n301 = global read "Meas_global.vi" "Duplicate channels"() -> (w610:i32[])
            n302 = case shown="True" "Select Duplicate Channels" {
              tunnel: w613 -> [_ _]
              tunnel: w611 -> [w621 w644]
              tunnel: w610 -> [w615 w637]
              tunnel: [w614 w636] -> w609
              frame False {
                n303 = for {
                  tunnel: w621 -> [w635] mode=indexing
                  tunnel: [w634] -> w622 mode=indexing
                  n304 = Unbundle By Name(w635) -> ("Inst type"=w634:T2)
                }
                n305 = for {
                  tunnel: w615 -> [w631] mode=indexing
                  tunnel: w622 -> [w633]
                  tunnel: [w632] -> w626 mode=indexing
                  tunnel: [w631] -> w623 mode=indexing
                  n306 = Index Array(array=w633, index=w631) -> (element=w632:T2)
                }
                n307 = Array Size(array=w621) -> (size(s)=w624:i32)
                n308 = Array Max & Min(array=w626) -> (max value=w627:T2, min value=w628:T2)  [unwired: 2 out]
                n309 = Array Max & Min(array=w623) -> (max index (indices)=w625:i32)  [unwired: 3 out]
                n310 = Array Size(array=w615) -> (size(s)=w620:i32)
                n311 = Equal?(x=w627, y=w628) -> (x = y?=w630:bool)
                n312 = Greater?(x=w620, y=1) -> (0:w617:bool)
                n313 = Greater?(x=w624, y=w625) -> (0:w629:bool)
                n314 = Compound Arithmetic op=AND(w617, w630, w629) -> (w616:bool)
                n315 = Select(t=w615, s=w616, f=i32[] [] ("32bit integer")) -> (s? t:f=w614:i32[])
              }
              frame True {
                n316 = for {
                  tunnel: w644 -> [w651] mode=indexing
                  shift-right: [w646] -> w640
                  shift-left: string[] [] -> [w647]
                  tunnel: w637 -> [w649]
                  tunnel: [w645] -> w639 mode=indexing
                  i -> [w650]
                  n317 = Unbundle By Name(w651) -> ("Inst name"=w645:string)
                  n318 = Search 1D Array(1D array=w649, element=w650) -> (index of element=w648:i32)  [unwired: 1 out]
                  n319 = case shown="0, Default" w648 {
                    tunnel: w647 -> [w654 w655]
                    tunnel: w645 -> [w653 _]
                    tunnel: [w652 w655] -> w646
                    frame 0, Default {
                      n320 = Build Array (concatenate)(w654, w653) -> (w652:string[])
                    }
                    frame -1 {
                    }
                  }
                }
                n321 = call "Select_Strings.vi"("Available Ch names"=w639, "Message"="Please select similar instruments whose results columns will be combined", "Selector mode"=T15."Zero or more", "Desired Ch names (in)"=w640) -> ("Ch Indicies Choosen"=w636:i32[])  [unwired: 4 out]
                n322 = local write "Select Duplicate Channels"(FALSE ("Select Local ADAM Channels")) -> ()
              }
            }
            n323 = global write "Meas_global.vi" "Duplicate channels"(w609) -> ()
          }
          frame #20 {
            n324 = local read "XW Present?"() -> (w658:bool)
            n325 = case shown="\"Take LDA data\"" "LDA data" {
              tunnel: [w667 w670] -> w660
              tunnel: w661 -> [_ w668]
              tunnel: w662 -> [_ _]
              tunnel: [w667 w669] -> w657
              frame "No LDA data" {
                w666 = FALSE  # Synchronise Analogue channels with LDA
                w667 = u8 2  # Disabled
                n326 = local write "Synchronise Analogue channels with LDA"(w666) -> ()
              }
              frame "Take LDA data" {
                n327 = stacked-sequence {
                  tunnel: [w671 _] -> w670
                  tunnel: [_ w673] -> w669
                  tunnel: w668 -> [_ w674]
                  frame #0 {
                    w671 = u8 0  # Disabled
                  }
                  frame #1 {
                    n328 = Array Size(array=w674) -> (size(s)=w675:i32)
                    n329 = Not Equal To 0?(x=w675) -> (x != 0?=w672:bool)
                    n330 = case shown="False" w672 {
                      tunnel: w672 -> [w677 _]
                      tunnel: [w676 w678] -> w673
                      frame False {
                        w676 = u8 2  # Disabled
                        n331 = local write "Synchronise Analogue channels with LDA"(w677) -> ()
                      }
                      frame True {
                        w678 = u8 0  # Disabled
                      }
                    }
                  }
                }
              }
            }
            n332 = property on="Cross wire/LDA" class="Enum (strict)"("Visible"=w658) -> ()  [unwired: 2 in, 2 out]
            n333 = case shown="True" w658 {
              tunnel: [w664 "Cross wire"] -> w656
              frame False {
                w664 = T7."2nd component as calculated"  # Cross wire/LDA
              }
              frame True {
              }
            }
            n334 = global write "Meas_global.vi" "Cross wire + or -ve"(w656) -> ()
            n335 = Wait (ms)(milliseconds to wait=u32 100) -> ()  [unwired: 1 out]
            n336 = property on="Synchronise Analogue channels with LDA" class="Bool (strict)"("Disabled"=w657) -> ()  [unwired: 2 in, 2 out]
            n337 = property on="LDA set up" class="Clust (strict)"("Disabled"=w660) -> ()  [unwired: 2 in, 2 out]
          }
          frame #21 {
            n338 = And(x=w684, y=w685) -> (x .and. y?=w683:bool)
            n339 = local read "Synchronise Analogue channels with LDA"() -> (w682:bool)
            n340 = while {
              shift-left: _ -> [w711]
              shift-right: [w712] -> w679
              tunnel: [w713] -> w681
              stop <- FALSE continue-if-true
              n341 = local read "Setup filename selector"() -> (w712:u16)
              n342 = Not Equal?(x=w712, y=w711) -> (x != y?=w713:bool)
            }
            n343 = case shown="True" w682 {
              tunnel: w686 -> [_ w697]
              tunnel: w683 -> [_ w696]
              frame False {
              }
              frame True {
                n344 = case shown="True" w696 {
                  tunnel: w697 -> [_ w700]
                  frame False {
                  }
                  frame True {
                    n345 = for {
                      tunnel: w700 -> [w709] mode=indexing
                      tunnel: [w702] -> w699 mode=indexing
                      n346 = Unbundle By Name(w709) -> ("Inst type"=w708:T2, "Symbol"=w706:string)
                      n347 = Equal?(x=w706, y="Sync") -> (x = y?=w704:bool)
                      n348 = Equal?(x=Inst_type."Raw voltage" ("Inst type"), y=w708) -> (x = y?=w703:bool)
                      n349 = And(x=w703, y=w704) -> (x .and. y?=w702:bool)
                    }
                    n350 = Or Array Elements(Boolean array=w699) -> (logical OR=w698:bool)
                    n351 = case shown="False" w698 {
                      frame False {
                        n352 = One Button Dialog(message="To Perform LDA Sync you must provide a Raw voltage channel having the symbol \"Sync\"") -> ()  [unwired: 2 out]
                      }
                      frame True {
                      }
                    }
                  }
                }
              }
            }
            n353 = case shown="True" w681 {
              tunnel: [FALSE ("exists?") w695] -> w680
              tunnel: w679 -> [_ w693]
              frame False {
              }
              frame True {
                n354 = local read "Setup Paths"() -> (w694:string[])
                n355 = Index Array(array=w694, index=w693) -> (element=w691:string)
                n356 = call "Setup_Filepath.vi"("Setup File Type"=Setup_Filetype."Measurement Setups", "Filename in"=w691) -> ("Filename Out"=w690:path)  [unwired: 1 out]
                n357 = call "Does_file_exist_(simple).vi"("Pathname"=w690) -> ("exists?"=w695:bool)
              }
            }
            n358 = local write "Read Setup File?"(w680) -> ()
            n359 = Current VI's Path() -> (path=w687:path)
            n360 = call "Close_Panel_and_Abort.vi"("Vi path"=w687, "stop"="stop") -> ()  [unwired: 1 out]
          }
        }
      }
    }
    frame #5 {
      n361 = local read "LDA data"() -> (w716:enum16{"No LDA data", "Take LDA data"})
      n362 = case shown="\"Take LDA data\"" w716 {
        tunnel: [FALSE ("Synchronise Analogue channels with LDA") "Synchronise Analogue channels with LDA"] -> w715
        frame "No LDA data" {
        }
        frame "Take LDA data" {
        }
      }
      n363 = global write "Meas_global.vi" "Synchronise with LDA"(w715) -> ()
      n364 = global write "Meas_global.vi" "LDA data"(w716) -> ()
      n365 = global write "Meas_global.vi" "LDA set up"("LDA set up") -> ()
    }
    frame #6 {
      n366 = stacked-sequence {
        seq-local: [_ w756 _ _] -> [_ _ _ w814]
        seq-local: [_ _ w782 _] -> [_ _ _ w813]
        seq-local: [w724 _ _ _] -> [_ _ _ w801]
        tunnel: w721 -> [w723 _ _ w805]
        tunnel: w720 -> [_ _ _ w804]
        tunnel: w719 -> [w722 _ _ _]
        frame #0 {
          n367 = local read "PWA Data"() -> (w725:T1)
          n368 = case shown="\"One Ch PWA\"" w725 {
            tunnel: ["" w734] -> w724
            tunnel: w723 -> [_ w733]
            tunnel: w722 -> [_ w729]
            frame "No PWA Data" {
            }
            frame "One Ch PWA" {
              n369 = Not Equal?(x="Calib_Setup.xls", y=w729) -> (x != y?=w728:bool)
              n370 = case shown="\"Setup Front Panel\"" w733 {
                tunnel: [w738 w741 w744 w747] -> w732
                tunnel: [w737 w740 w743 w746] -> w731
                tunnel: [w736 w739 w742 w745] -> w727
                tunnel: w728 -> [w736 w739 w742 _]
                frame "Show Setup" {
                  w738 = TRUE  # Show Panel?
                  w737 = T4 FALSE  # OK
                }
                frame "Run Program" {
                  w741 = FALSE  # Show Panel?
                  w740 = T4 TRUE  # OK
                }
                frame "Save Current Setup" {
                  w744 = FALSE  # Show Panel?
                  w743 = T4 TRUE  # OK
                }
                frame "Setup Front Panel" {
                  w745 = FALSE  # Check Calib file?
                  w747 = FALSE  # Show Panel?
                  w746 = T4 TRUE  # OK
                }
              }
              n371 = global read "Meas_global.vi" "Pre Setup String"() -> (w735:string)
              n372 = call "PWA_Setup_Panel.vi"("Show Panel?"=w732, "Check Calib file?"=w727, "OK"=w731, "Incoming Setup String"=w735) -> ("Outgoing Setup String"=w734:string)  [unwired: 3 out]
            }
          }
        }
        frame #1 {
          n373 = local read "LDA set up"() -> (w761:T6)
          n374 = global read "Meas_global.vi" "Duplicate channels"() -> (w760:i32[])
          n375 = Unbundle By Name(w761) -> ("dimensions"=w753:enum16{"1D", "2D"}, "Analogue Freq Multiplier"=w751:dbl)
          n376 = case shown="\"2D\"" w753 {
            tunnel: ["1D" "2D"] -> w755
            frame "1D" {
            }
            frame "2D" {
            }
          }
          n377 = for {
            shift-right: [w764] -> w758
            shift-left: "" -> [w767]
            tunnel: w760 -> [w768] mode=indexing
            n378 = Number To Decimal String(number=w768) -> (decimal integer string=w766:string)  [unwired: 1 out]
            n379 = Concatenate Strings(w767, w766, "; ") -> (w764:string)
          }
          n380 = call "Characters_to_string.vi"("Characters to write"=w755, "Label for characters"="LDA Dimensions") -> ("Output string"=w754:string)
          n381 = call "Value_to_string.vi"("Value"=w751, "Label for value"="LDA Analog Freq Multiplier") -> ("Output string"=w748:string)  [unwired: 1 in]
          n382 = call "Characters_to_string.vi"("Characters to write"=w758, "Label for characters"="Log_Similar_Measurements_in_the _same_column") -> ("Output string"=w749:string)
          n383 = Concatenate Strings(w754, w748, w749) -> (w756:string)
        }
        frame #2 {
          n384 = global write "Meas_global.vi" "Trigger mode"("Trigger mode") -> ()
          n385 = local read "Cross wire"() -> (w785:T7)
          n386 = global read "Preference_global.vi" "Rig Setup"() -> (w771:string)
          n387 = Match Pattern(string=w771, regular expression="-") -> (before substring=w770:string)  [unwired: 4 out]
          n388 = case shown="\"Free Running\"" "Trigger mode" {
            tunnel: ["Free Running" "Trigger Every Block" "Trigger Every Sample" "Start on Trigger"] -> w780
            frame "Free Running" {
            }
            frame "Trigger Every Block" {
            }
            frame "Trigger Every Sample" {
            }
            frame "Start on Trigger" {
            }
          }
          n389 = property on="PWA Data" class="Enum (strict)"() -> ("Strings []"=w776:string[])  [unwired: 2 in, 2 out]
          n390 = global write "Meas_global.vi" "PWA Data"("PWA Data") -> ()
          n391 = Equal?(x=T7."2nd component multipled by -1" ("Cross wire/LDA"), y=w785) -> (x = y?=w784:bool)
          n392 = case shown="\"EnFlo_Tunnel\"" w770 {
            tunnel: ["" w792] -> w769
            frame "False", Default {
            }
            frame "EnFlo_Tunnel" {
              n393 = call "Characters_to_string.vi"("Characters to write"="FALSE", "Label for characters"="Show_all_EnFlo_Tunnel_Columns") -> ("Output string"=w792:string)
            }
          }
          n394 = Index Array(array=w776, index="PWA Data") -> (element=w775:string)
          n395 = Select(t="TRUE", s=w784, f="FALSE") -> (s? t:f=w787:string)
          n396 = call "Characters_to_string.vi"("Characters to write"=w775, "Label for characters"="Pulsed_Wire_Data" ("Variable name")) -> ("Output string"=w774:string)
          n397 = call "Characters_to_string.vi"("Characters to write"=w787, "Label for characters"="Invert Second Component") -> ("Output string"=w783:string)
          n398 = call "Characters_to_string.vi"("Characters to write"=w780, "Label for characters"="Trigger mode") -> ("Output string"=w778:string)
          n399 = Concatenate Strings(w778, w774, w783, w769) -> (w782:string)
        }
        frame #3 {
          w806 = FALSE  # Show Panel?
          n400 = for {
            tunnel: w804 -> [w819] mode=indexing
            tunnel: [w818] -> w800 mode=indexing
            n401 = Unbundle By Name(w819) -> ("Ch Name"=w818:string)
          }
          n402 = global read "Meas_global.vi" "Pre Setup String"() -> (w807:string)
          n403 = call "Choose_Plug_In_to_Run.vi"("setup"=w805, "Show Panel?"=w806, "Setup String In"=w807) -> ("Setup String Out"=w808:string)  [unwired: 1 out]
          n404 = Array To Spreadsheet String(array=w800, 3:"%s" ("format string")) -> (spreadsheet string=w802:string)  [unwired: 1 out]
          n405 = call "Add_label_to_string.vi"("String to write"=w802, "File Label"="Local ADAM Channels") -> ("Output string"=w815:string)
          n406 = call "Date_and_Time_to_string.vi"() -> ("Date and time (spreadsheet)"=w810:string)
          n407 = global read "Meas_global.vi" "New Setup String"() -> (w809:string)
          n408 = call "Value_to_string.vi"("Value"="Sync Delay Time (ms)", "Label for value"="Sync Delay Time (ms)" ("Label for characters")) -> ("Output string"=w803:string)  [unwired: 1 in]
          n409 = Concatenate Strings(w809, w801, w808, w810, w814, w813, w815, w803) -> (w817:string)
          n410 = global write "Meas_global.vi" "New Setup String"(w817) -> ()
          n411 = global write "LDA_meas_global_1.vi" "Sync Delay Time (ms)"("Sync Delay Time (ms)") -> ()
        }
      }
    }
    frame #7 {
      n412 = case shown="\"Take New Data\"" w822 {
        tunnel: w821 -> [w829 w864]
        tunnel: [w823 w858] -> w820
        frame "Take New Data" {
          n413 = for {
            tunnel: w829 -> [w840] mode=indexing
            shift-right: [w836] -> w826
            shift-left: i16[] [] -> [w838]
            shift-right: [w834] -> w825
            shift-left: path[] [] -> [w835]
            tunnel: [w831] -> w823 mode=indexing
            n414 = Unbundle By Name(w840) -> ("Use Latest"=w833:bool, "Inst type"=w839:T2, "Ch No"=w837:i16, "Calib filename"=w832:path)
            n415 = call "Current_Filepath.vi"("Filename in"=w832, "Data Type"="Calibrations") -> ("Filename Out"=w831:path)  [unwired: 1 out]
            n416 = case shown="\"Propeller anemometer\", Default" w839 {
              tunnel: w838 -> [w847 w857]
              tunnel: w837 -> [w846 _]
              tunnel: [w845 w857] -> w836
              tunnel: w835 -> [w844 w856]
              tunnel: w832 -> [w843 _]
              tunnel: [w842 w856] -> w834
              tunnel: w833 -> [w841 _]
              frame "Propeller anemometer", Default {
                n417 = case shown="False" w841 {
                  tunnel: w847 -> [w853 w855]
                  tunnel: w846 -> [w852 _]
                  tunnel: [w851 w855] -> w845
                  tunnel: w844 -> [w850 w854]
                  tunnel: w843 -> [w849 _]
                  tunnel: [w848 w854] -> w842
                  frame False {
                    n418 = Build Array (concatenate)(w853, w852) -> (w851:i16[])
                    n419 = Build Array (concatenate)(w850, w849) -> (w848:path[])
                  }
                  frame True {
                  }
                }
              }
              frame "Raw voltage" {
              }
            }
          }
          n420 = call "Current_Calib_Filenames.vi"("Calib Filename"=w825, "Channel Numbers"=w826, "Mode"=App_Global."Write to Global") -> ()  [unwired: 3 out]
        }
        frame "Post Process Raw Data File" {
          n421 = for {
            tunnel: w864 -> [w870] mode=indexing
            tunnel: [w869] -> w858 mode=indexing
            n422 = Unbundle By Name(w870) -> ("Calib filename"=w869:path)
          }
          n423 = global read "Meas_global.vi" "Pre Setup String"() -> (w863:string)
          n424 = call "Get_Characters_from_string.vi"("Input string"=w863, "Variable name"="Skip_Block_Numbers_(eg 1;2;5;12)") -> ("Status"=w861:enum16{"Char in string", "Char not in string"}, "Value"=w860:string)  [unwired: 1 in]
          n425 = case shown="\"Char in string\"" w861 {
            tunnel: w860 -> [w867 _]
            tunnel: [w865 i32[] []] -> w859
            frame "Char in string" {
              n426 = call "Get_array_values_fr_String.vi"("String Value"=w867) -> ("Numeric Array"=w866:dbl[])  [unwired: 1 out]
              n427 = To Long Integer(number=w866) -> (32bit integer=w865:i32[])
            }
            frame "Char not in string" {
            }
          }
          n428 = global write "Meas_global.vi" "Blocks to Skip"(w859) -> ()
        }
      }
    }
    frame #8 {
      n429 = global read "Meas_global.vi" "Pre Setup String"() -> (w871:string)
      n430 = for {
        tunnel: [w882] -> w874 mode=indexing
        tunnel: w873 -> [w879] mode=indexing
        tunnel: w872 -> [w881] mode=indexing
        tunnel: w871 -> [w880]
        n431 = Unbundle By Name(w879) -> ("Code name"=w878:string)
        n432 = Concatenate Strings(w878, "_Av_SamplingRate" ("string")) -> (w876:string)
        n433 = call "Get_value_from_string.vi"("Input string"=w880, "Variable name"=w876) -> ("Value"=w875:dbl)  [unwired: 1 in, 1 out]
        n434 = Bundle By Name(cluster=w879, "Calib File"=w881, "Av Sampling Rate"=w875) -> (w882:T8)
      }
      "Analysis Info cluster" <- w874
    }
  }
